vi "String Split at Count.vi"(2 "# of characters in 1st string":i32, 3 "String to Split":string) -> (0 "2nd String":string, 1 "1st String":string)   [LabVIEW 2020, in "Associated Research 78XX Series.lvlib"]
uses:
  <instrlib>/Associated Research 78XX Series/Associated Research 78XX Series.lvlib
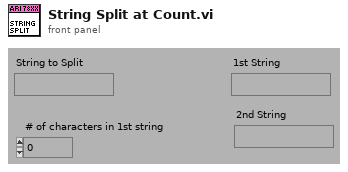
[diagram p1: front panel]
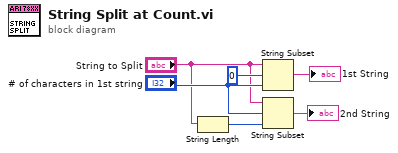
[diagram p0: block diagram]
diagram:
  n1 = String Length(string="String to Split") -> (length=w3:i32)
  n2 = String Subset(string="String to Split", offset (0)=0, length (rest)="# of characters in 1st string") -> (substring=→"1st String":string)
  n3 = String Subset(string="String to Split", offset (0)="# of characters in 1st string", length (rest)=w3) -> (substring=→"2nd String":string)
